vi "Provider_OnPopupMenu.vi"(11 "objects":T1[](array[typedef])) -> ()   [LabVIEW 2020, in "Message Maker Provider.lvlib"]
uses:
  Message Maker Provider.lvlib
  <resource>/Framework/Providers/API/mxLvMenuItem.ctl
  Support/Localized Strings.vi
  AFPP Shared/Validation Mode.ctl
  AFPP Shared/AFPP Shared.lvlib
  <resource>/Framework/Providers/API/ItemRef.ctl
panel:
  out "error out":errorcluster
  in  "error in":errorcluster
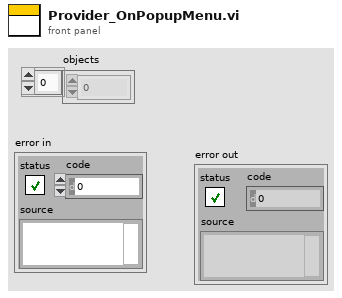
[diagram p1: front panel]
types:
  T1 = typedef "ItemRef.ctl" = u64
  T2 = typedef "AFPP Shared.lvlib/Validation Mode.ctl" = enum16{"An Actor Library", "A Target Tag"}
  T3 = typedef "mxLvMenuItem.ctl" = cluster{"Menu Name":string, "Description":string, "Icon File Name":path, "Menu Tag":string, "Enabled":bool, "Checked":bool, "Separator":bool, "Batchable":bool, "Weight":i32, "Batch Mode (Ignored if Not Batchable)":enum32{"Show If All Items Support Command", "Show If Any Items Support Command"}, "Menu Location":enum32{"<None>", "Project", "Project / Build Specifications", "Tools", "Tools / Source Control", "Tools / Real-Time Module", "Help"}, "Exclude From Getting Started Window Menu":bool}
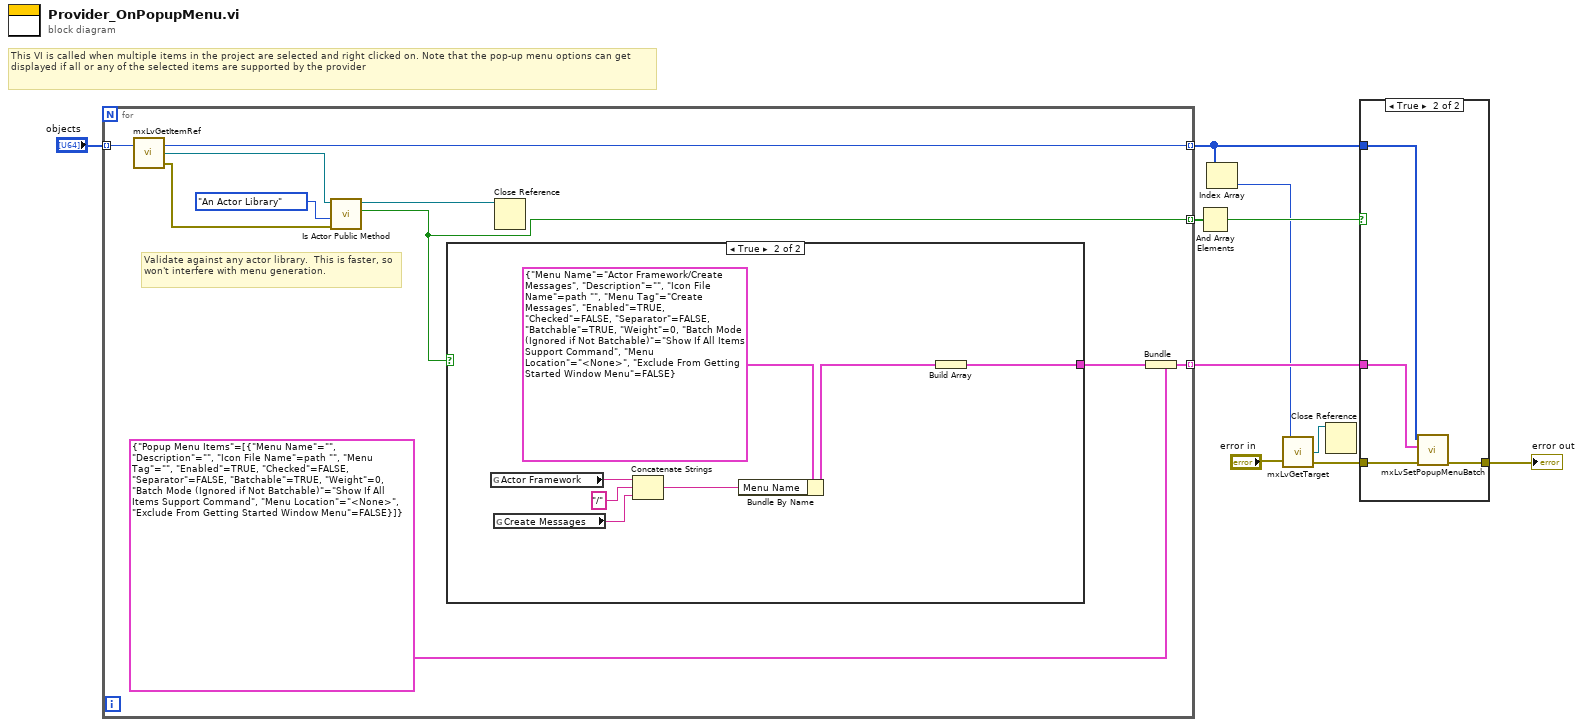
[diagram p0: block diagram]
diagram:
  # "This VI is called when multiple items in the project are selected and right clicked on. Note that the pop-up menu options can get displayed if all or any of the selected items are supported by the provider"
  n1 = for {
    tunnel: [w20] -> w10 mode=indexing
    tunnel: "objects" -> [w19] mode=indexing
    tunnel: [w18] -> w2 mode=indexing
    tunnel: [w13] -> w7 mode=indexing
    # "Validate against any actor library.  This is faster, so won't interfere with menu generation."
    n2 = call <resource>:"mxLvGetItemRef.vi"("Item"=w19) -> ("Item"=w18:T1, "Item Refnum"=w15:refnum<vi>, "error out"=w14:errorcluster)  [unwired: 1 in]
    n3 = call "Is Actor Public Method.vi"("error in (no error)"=w14, "Validation"=Validation_Mode."An Actor Library", "ProjectItem in"=w15) -> ("Is Actor Public Method"=w13:bool, "ProjectItem out"=w16:refnum<vi>)  [unwired: 5 in, 2 out]
    n4 = case shown="True" w13 {
      tunnel: [_ w21] -> w12
      frame False {
      }
      frame True {
        n5 = global read "Localized Strings.vi" "Actor Framework"() -> (w25:string)
        n6 = global read "Localized Strings.vi" "Create Messages"() -> (w22:string)
        n7 = Concatenate Strings(w25, "/", w22) -> (w24:string)
        n8 = Bundle By Name(cluster=T3 {"Menu Name"="Actor Framework/Create Messages", "Description"="", "Icon File Name"=path "", "Menu Tag"="Create Messages", "Enabled"=TRUE, "Checked"=FALSE, "Separator"=FALSE, "Batchable"=TRUE, "Weight"=0, "Batch Mode (Ignored if Not Batchable)"=enum."Show If All Items Support Command", "Menu Location"=enum."<None>", "Exclude From Getting Started Window Menu"=FALSE} ("Menu Item"), "Menu Name"=w24) -> (w26:T3)
        n9 = Build Array(w26) -> (w21:T3[])
      }
    }
    n10 = Close Reference(reference=w16) -> ()  [unwired: 1 in, 1 out]
    n11 = Bundle(cluster=cluster{"Popup Menu Items":T3[]} {"Popup Menu Items"=[{"Menu Name"="", "Description"="", "Icon File Name"=path "", "Menu Tag"="", "Enabled"=TRUE, "Checked"=FALSE, "Separator"=FALSE, "Batchable"=TRUE, "Weight"=0, "Batch Mode (Ignored if Not Batchable)"=enum."Show If All Items Support Command", "Menu Location"=enum."<None>", "Exclude From Getting Started Window Menu"=FALSE}]}, "Popup Menu Items"=w12) -> (w20:cluster{"Popup Menu Items":T3[]})
  }
  n12 = And Array Elements(Boolean array=w7) -> (logical AND=w6:bool)
  n13 = Index Array(array=w2) -> (element=w1:T1)  [unwired: 1 in]
  n14 = call <resource>:"mxLvGetTarget.vi"("Item"=w1, "error in"="error in") -> ("Target"=w5:refnum<vi>, "error out"=w4:errorcluster)  [unwired: 1 out]
  n15 = Close Reference(reference=w5) -> ()  [unwired: 1 in, 1 out]
  n16 = case shown="True" w6 {
    tunnel: w10 -> [_ w32]
    tunnel: [w28 w31] -> w9
    tunnel: w4 -> [w28 w30]
    tunnel: w2 -> [_ w29]
    frame False {
    }
    frame True {
      n17 = call <resource>:"mxLvSetPopupMenuBatch.vi"("error in"=w30, "Menu Items"=w32, "Items"=w29) -> ("error out"=w31:errorcluster)  [unwired: 7 in, 1 out]
    }
  }
  "error out" <- w9
